vi "StraightCurveY.vi"(11 "9dots":dbl[][](array[numeric])) -> (3 "曲面调整":dbl)   [LabVIEW 2011]
uses:
  <vilib>/vision/NI_Vision_Development_Module.lvlib
  <vilib>/Analysis/NI_AALBase.lvlib
panel:
  out "Distances":sgl[](array[numeric]) format="%.4f"
  out "Distances 2":sgl[](array[numeric]) format="%.4f"
  out "Distances 3":sgl[](array[numeric]) format="%.4f"
  out "r":dbl
  out "detaY":dbl caption="均值" format="%0.2f"
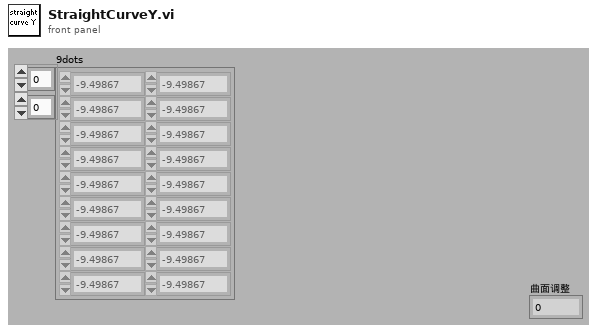
[diagram p1: front panel]
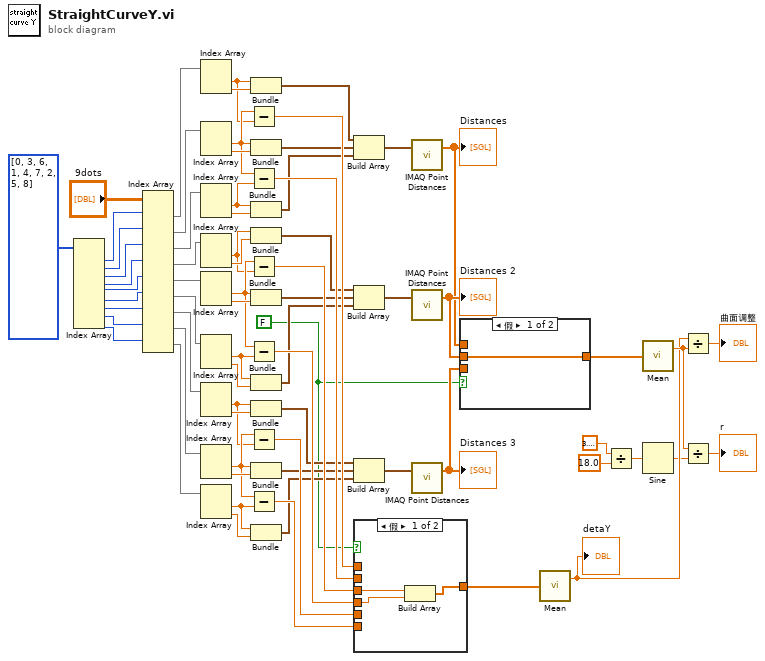
[diagram p0: block diagram]
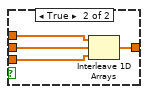
[diagram p2: hidden frame]
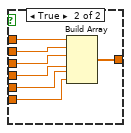
[diagram p3: hidden frame]
diagram:
  w1 = FALSE
  n1 = Index Array(array=i32[] [0, 3, 6, 1, 4, 7, 2, 5, 8] ("Distances 4")) -> (element #1=w20:i32, element #2=w19:i32, element #3=w18:i32, element #4=w17:i32, element #5=w16:i32, element #6=w15:i32, element #7=w14:i32, element #8=w13:i32, element #9=w12:i32)  [unwired: 9 in]
  n2 = Index Array(array="9dots", index (row) #1=w20, index (row) #2=w19, index (row) #3=w18, index (row) #4=w17, index (row) #5=w16, index (row) #6=w15, index (row) #7=w14, index (row) #8=w13, index (row) #9=w12) -> (element #1=w22:dbl[], element #2=w23:dbl[], element #3=w24:dbl[], element #4=w25:dbl[], element #5=w26:dbl[], element #6=w27:dbl[], element #7=w28:dbl[], element #8=w29:dbl[], element #9=w30:dbl[])  [unwired: 9 in]
  n3 = Index Array(array=w22) -> (element #1=w9:dbl, element #2=w52:dbl)  [unwired: 2 in]
  n4 = Index Array(array=w23) -> (element #1=w10:dbl, element #2=w51:dbl)  [unwired: 2 in]
  n5 = Index Array(array=w24) -> (element #1=w8:dbl, element #2=w53:dbl)  [unwired: 2 in]
  n6 = Index Array(array=w25) -> (element #1=w6:dbl, element #2=w55:dbl)  [unwired: 2 in]
  n7 = Index Array(array=w26) -> (element #1=w7:dbl, element #2=w54:dbl)  [unwired: 2 in]
  n8 = Index Array(array=w27) -> (element #1=w5:dbl, element #2=w56:dbl)  [unwired: 2 in]
  n9 = Index Array(array=w28) -> (element #1=w3:dbl, element #2=w57:dbl)  [unwired: 2 in]
  n10 = Index Array(array=w29) -> (element #1=w4:dbl, element #2=w65:dbl)  [unwired: 2 in]
  n11 = Index Array(array=w30) -> (element #1=w2:dbl, element #2=w58:dbl)  [unwired: 2 in]
  n12 = Subtract(x=w10, y=w9) -> (x-y=w59:dbl)
  n13 = Subtract(x=w10, y=w8) -> (x-y=w60:dbl)
  n14 = Subtract(x=w7, y=w6) -> (x-y=w61:dbl)
  n15 = Subtract(x=w7, y=w5) -> (x-y=w62:dbl)
  n16 = Subtract(x=w4, y=w3) -> (x-y=w63:dbl)
  n17 = Subtract(x=w4, y=w2) -> (x-y=w64:dbl)
  n18 = Bundle("Numeric"=w9, "Numeric"=w52) -> (w31:cluster{"Numeric":dbl, "Numeric":dbl})  [unwired: 1 out]
  n19 = Bundle("Numeric"=w10, "Numeric"=w51) -> (w32:cluster{"Numeric":dbl, "Numeric":dbl})  [unwired: 1 out]
  n20 = Bundle("Numeric"=w8, "Numeric"=w53) -> (w33:cluster{"Numeric":dbl, "Numeric":dbl})  [unwired: 1 out]
  n21 = Bundle("Numeric"=w6, "Numeric"=w55) -> (w34:cluster{"Numeric":dbl, "Numeric":dbl})  [unwired: 1 out]
  n22 = Bundle("Numeric"=w7, "Numeric"=w54) -> (w35:cluster{"Numeric":dbl, "Numeric":dbl})  [unwired: 1 out]
  n23 = Bundle("Numeric"=w5, "Numeric"=w56) -> (w36:cluster{"Numeric":dbl, "Numeric":dbl})  [unwired: 1 out]
  n24 = Bundle("Numeric"=w3, "Numeric"=w57) -> (w37:cluster{"Numeric":dbl, "Numeric":dbl})  [unwired: 1 out]
  n25 = Bundle("Numeric"=w4, "Numeric"=w65) -> (w38:cluster{"Numeric":dbl, "Numeric":dbl})  [unwired: 1 out]
  n26 = Bundle("Numeric"=w2, "Numeric"=w58) -> (w39:cluster{"Numeric":dbl, "Numeric":dbl})  [unwired: 1 out]
  n27 = Build Array(w31, w32, w33) -> (w40:cluster{"Numeric":dbl, "Numeric":dbl}[])
  n28 = Build Array(w34, w35, w36) -> (w41:cluster{"Numeric":dbl, "Numeric":dbl}[])
  n29 = Build Array(w37, w38, w39) -> (w42:cluster{"Numeric":dbl, "Numeric":dbl}[])
  n30 = case shown="假" w1 {
    tunnel: [w71 w80] -> w66
    tunnel: w64 -> [_ w79]
    tunnel: w63 -> [_ w78]
    tunnel: w62 -> [w72 w77]
    tunnel: w61 -> [w73 w76]
    tunnel: w60 -> [_ w75]
    tunnel: w59 -> [_ w74]
    frame False {
      n31 = Build Array(w73, w72) -> (w71:dbl[])
    }
    frame True {
      n32 = Build Array(w74, w75, w76, w77, w78, w79) -> (w80:dbl[])
    }
  }
  n33 = call "IMAQ Point Distances"("Points"=w40) -> ("Distances"=w43:sgl[])  [unwired: 1 in, 4 out]
  "Distances" <- w43
  n34 = call "IMAQ Point Distances"("Points"=w41) -> ("Distances"=w44:sgl[])  [unwired: 1 in, 4 out]
  "Distances 2" <- w44
  n35 = call "IMAQ Point Distances"("Points"=w42) -> ("Distances"=w45:sgl[])  [unwired: 1 in, 4 out]
  "Distances 3" <- w45
  n36 = case shown="假" w1 {
    tunnel: [w81 w85] -> w46
    tunnel: w45 -> [_ w84]
    tunnel: w44 -> [w81 w83]
    tunnel: w43 -> [_ w82]
    frame False {
    }
    frame True {
      n37 = Interleave 1D Arrays(w82, w83, w84) -> (w85:sgl[])
    }
  }
  n38 = call <vilib>:"Mean.vi"("X"=w66) -> ("mean"=w67:dbl)  [unwired: 1 out]
  "detaY" <- w67
  n39 = Divide(x=3.141592653589793, y=18.0) -> (x/y=w50:dbl)
  n40 = call <vilib>:"Mean.vi"("X"=w46) -> ("mean"=w69:dbl)  [unwired: 1 out]
  n41 = Sine(x=w50) -> (sin(x)=w47:dbl)
  n42 = Divide(x=w67, y=w69) -> (x/y=→"曲面调整":dbl)
  n43 = Divide(x=w69, y=w47) -> (x/y=→"r":dbl)
